vi "fun_XY2RPhase.vi"(8 "error in (no error)":errorcluster, 9 "Preset":u16, 10 "Demod Sample Out":T1) -> (0 "error out":errorcluster, 1 "Y or Phase":dbl, 2 "X or R":dbl, 3 "waveform (Y)":waveform(dbl)[](array[waveform]))   [LabVIEW 2016]
uses:
  <instrlib>/Zurich Instruments LabOne/Public/Data/ziTypeDemodSampleSingle.ctl
  <instrlib>/Zurich Instruments LabOne/Zurich Instruments LabOne.lvlib
panel:
  out "waveform Y or Phase":waveform(dbl)
  out "waveform X or R":waveform(dbl)
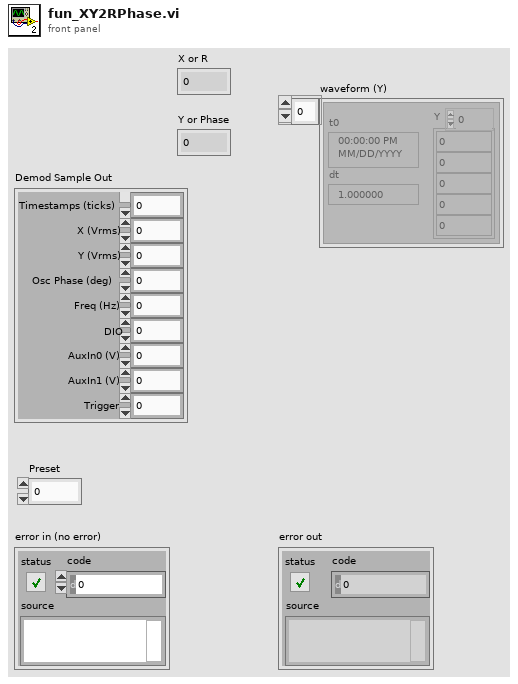
[diagram p1: front panel]
types:
  T1 = typedef "Zurich Instruments LabOne.lvlib/ziTypeDemodSampleSingle.ctl" = cluster{"Timestamps (ticks)":u64, "X (Vrms)":dbl, "Y (Vrms)":dbl, "Osc Phase (deg)":dbl, "Freq (Hz)":dbl, "DIO":u32, "AuxIn0 (V)":dbl, "AuxIn1 (V)":dbl, "Trigger":u32}
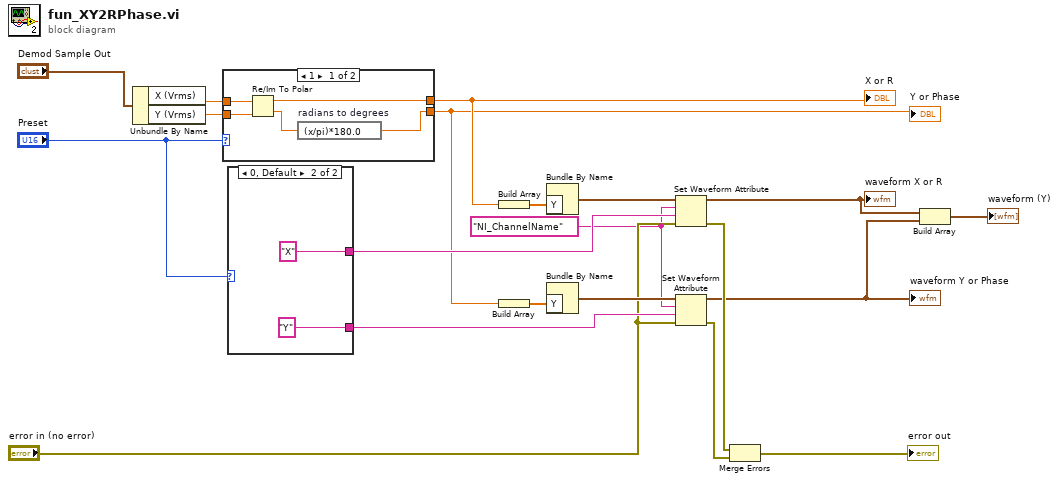
[diagram p0: block diagram]
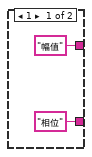
[diagram p2: hidden frame]
diagram:
  w2 = "NI_ChannelName" ("name")
  n1 = Unbundle By Name("Demod Sample Out") -> ("X (Vrms)"=w19:dbl, "Y (Vrms)"=w20:dbl)
  n2 = case shown="1" "Preset" {
    tunnel: w19 -> [w25 w27]
    tunnel: [w24 w27] -> w16
    tunnel: [w21 w26] -> w11
    tunnel: w20 -> [w23 w26]
    frame 1 {
      n3 = Re/Im To Polar(2:w23, 3:w25) -> (0:w22:dbl, 1:w24:dbl)
      n4 = expression code="(x/pi)*180.0" "radians to degrees"(w22) -> (w21:dbl)
    }
    frame 0, Default {
    }
  }
  "Y or Phase" <- w11
  "X or R" <- w16
  n5 = case shown="0, Default" "Preset" {
    tunnel: ["幅值" "X"] -> w14
    tunnel: ["相位" "Y"] -> w10
    frame 1 {
    }
    frame 0, Default {
    }
  }
  n6 = Build Array(w16) -> (w17:dbl[])
  n7 = Build Array(w11) -> (w12:dbl[])
  n8 = Bundle By Name("Y"=w17) -> (w15:waveform(dbl))  [unwired: 1 in]
  n9 = Bundle By Name("Y"=w12) -> (w13:waveform(dbl))  [unwired: 1 in]
  n10 = Set Waveform Attribute(4:"error in (no error)", 5:w14, 6:w2, 7:w15) -> (0:w8:errorcluster, 3:w5:waveform(dbl))  [unwired: 1 out]
  "waveform X or R" <- w5
  n11 = Set Waveform Attribute(4:"error in (no error)", 5:w10, 6:w2, 7:w13) -> (0:w7:errorcluster, 3:w4:waveform(dbl))  [unwired: 1 out]
  "waveform Y or Phase" <- w4
  n12 = Merge Errors(w8, w7) -> (→"error out":errorcluster)
  n13 = Build Array(w5, w4) -> (→"waveform (Y)":waveform(dbl)[])
